vi "Set Multiple Endpoint Configurations.vi"(8 "error in":errorcluster, 10 "endpoint configurations":T1[](array[typedef]), 11 "endpoint configuration in":T3 format="%.0x") -> (0 "error out":errorcluster, 3 "endpoint configuration out":T3 format="%.0x")   [LabVIEW 2020, in "SLSC Switch Scripting.lvlib"]
doc: "Sets the configuration for multiple endpoints. This is faster than calling <b>Set Endpoint Configuration.vi</b> multiple times."
uses:
  SLSC Switch Scripting.lvlib
  <vilib>/NI VeriStand/Custom Device API/Custom Device Item Ref.ctl
  Shared/Endpoint Configuration Cluster.ctl
  Shared/Endpoint Configuration Enum.ctl
  <vilib>/NI VeriStand/Custom Device API/Custom Device API.lvlib
  Dependencies.llb/SLSC Switch Shared.lvlib
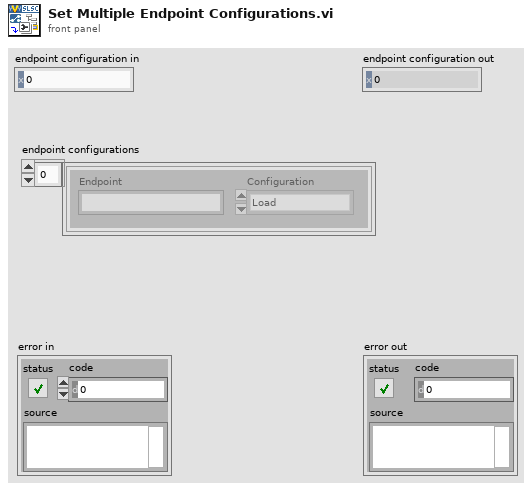
[diagram p1: front panel]
types:
  T1 = typedef "SLSC Switch Shared.lvlib/Endpoint Configuration Cluster.ctl" = cluster{"Endpoint":string, "Configuration":T2}
  T2 = typedef "SLSC Switch Shared.lvlib/Endpoint Configuration Enum.ctl" = enum16{"Load", "Source", "Configuration"}
  T3 = typedef "Custom Device API.lvlib/Custom Device Item Ref.ctl" = u64
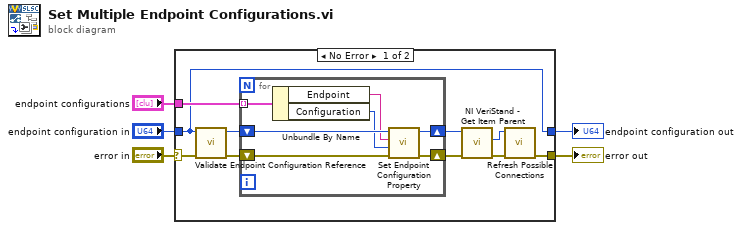
[diagram p0: block diagram]
diagram:
  n1 = case shown="No Error" "error in" {
    selector: "error in" -> [w15 w24]
    tunnel: "endpoint configurations" -> [w14 _]
    tunnel: [w8 w24] -> w3
    tunnel: "endpoint configuration in" -> [w6 w23]
    tunnel: [w6 w23] -> w1
    frame No Error {
      n2 = call "Validate Endpoint Configuration Reference.vi"("error in"=w15, "endpoint configuration in"=w6) -> ("error out"=w13:errorcluster, "endpoint configuration out"=w12:T3)  [unwired: 8 in]
      n3 = for {
        shift-right: [w19] -> w9
        shift-left: w13 -> [w20]
        shift-right: [w21] -> w7
        shift-left: w12 -> [w22]
        tunnel: w14 -> [w18] mode=indexing
        n4 = Unbundle By Name(w18) -> ("Endpoint"=w17:string, "Configuration"=w16:T2)
        n5 = call "Set Endpoint Configuration Property.vi"("error in"=w20, "configuration"=w16, "endpoint"=w17, "endpoint configuration in"=w22) -> ("error out"=w19:errorcluster, "endpoint configuration out"=w21:T3)  [unwired: 6 in]
      }
      n6 = call <vilib>:"NI VeriStand - Get Item Parent.vi"("error in (no error)"=w9, "Item Ref in"=w7) -> ("error out"=w10:errorcluster, "Parent Ref"=w11:T3)  [unwired: 6 in, 2 out]
      n7 = call "Refresh Possible Connections.vi"("error in"=w10, "slsc switch custom device in"=w11) -> ("error out"=w8:errorcluster)  [unwired: 8 in, 1 out]
    }
    frame Error {
    }
  }
  "error out" <- w3
  "endpoint configuration out" <- w1
